vi "State_Machine.vi"(8 "error in (no error)":errorcluster caption="entrée d'erreur (pas d'erreur)", 11 "Send_Frame en entrée":refnum<class "Zigbee_Send_Command_UART.lvclass">) -> (0 "error out":errorcluster caption="sortie d'erreur", 2 "Json_String":string, 3 "Send_Frame en sortie":refnum<class "Zigbee_Send_Command_UART.lvclass">)   [LabVIEW 2020, in "Library Test.lvlib" / "Zigbee_Send_Command_UART.lvclass"]
uses:
  Zigbee_Send_Command_UART.lvclass
  Commun VI/TypeDef/Liste Error.ctl
  Zigbee_Send_Command_UART.lvclass/Zigbee_Send_Command_UART.ctl
  Commun VI/Library Commun.lvlib
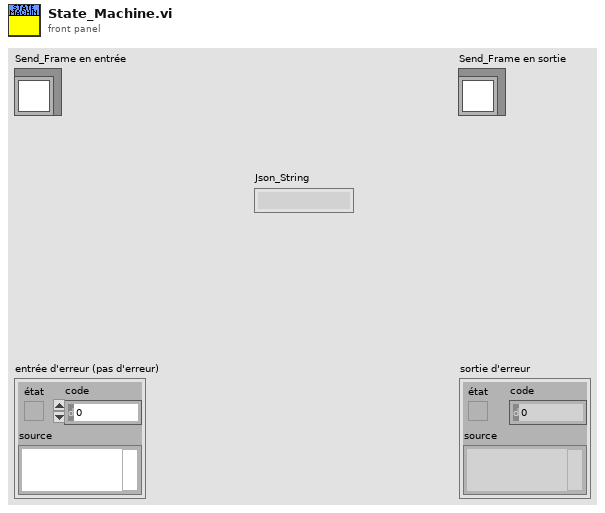
[diagram p1: front panel]
types:
  T1 = enum16{"Empty port", "Send Frame", "Wait Return", "Check End", "End"}
  T2 = typedef "Library Commun.lvlib/Liste Error.ctl" = enum16{"Firebase Driver - Get Document", "Firebase Driver - Get Document With Where", "Firebase Driver - Delete Document", "Firebase Driver - Set Document", "Firebase Driver - Update Document", "Firebase Altyor - Search Document Bench", "Firebase Altyor - Class Not in Firebase", "Spectrum_Analyser - Timeout", "Relay Board - Qty Relay", "DIO - Pb Funtion", "Power_Supply - Peripherical not find", "Mutimeter - Peripherical not find", "Instrument - Function Not Used", "Instrument - Instrument name not specified", "Instrument - Allready Initialised", "Instrument - TimeOut", "Instrument - the instrument must be Initialise before", "Instrument - Frame Not received", "Instrument - Frame Nok", "Test - Initialise the File_for_Save", "Test - Timeout", "Test - Cmd Error", "FGV - Variable ", "BDD FireBase - Define Class", "SN - Class Not Define"}
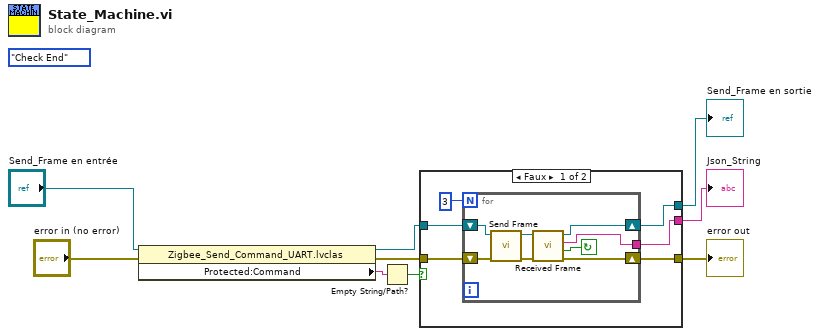
[diagram p0: block diagram]
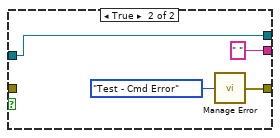
[diagram p2: hidden frame]
diagram:
  (unwired) T1."Check End"
  n1 = property class="Zigbee_Send_Command_UART.lvclas"(reference="Send_Frame en entrée", error in="error in (no error)") -> (reference out=w8:refnum<class "Zigbee_Send_Command_UART.lvclass">, error out=w7:errorcluster, "Protected:Command"=w4:string)
  n2 = Empty String/Path?(string/path=w4) -> (empty?=w3:bool)
  n3 = case shown="Faux" w3 {
    tunnel: [w13 w25] -> w2
    tunnel: w8 -> [w15 w25]
    tunnel: w7 -> [w14 _]
    tunnel: [w12 w27] -> w5
    tunnel: [w10 " " ("Frame read")] -> w1
    frame False {
      n4 = for {
        N: 3 -> [_]
        shift-right: [w20] -> w13
        shift-left: w15 -> [w23]
        shift-right: [w18] -> w12
        shift-left: w14 -> [w22]
        tunnel: [w16] -> w10
        stop <- w17 continue-if-true
        n5 = call-dynamic "Send Frame.vi"("entrée d'erreur (pas d'erreur)"=w22, "Send_Frame en entrée"=w23) -> ("sortie d'erreur"=w19:errorcluster, "Send_Frame en sortie"=w21:refnum<class "Zigbee_Send_Command_UART.lvclass">)  [unwired: 8 in]
        n6 = call-dynamic "Received Frame.vi"("entrée d'erreur (pas d'erreur)"=w19, "Send_Frame en entrée"=w21) -> ("sortie d'erreur"=w18:errorcluster, "Send again"=w17:bool, "Frame read"=w16:string, "Send_Frame en sortie"=w20:refnum<class "Zigbee_Send_Command_UART.lvclass">)  [unwired: 6 in]
      }
    }
    frame True {
      n7 = call "Manage Error.vi"("Code Erreur"=Liste_Error."Test - Cmd Error") -> ("error out"=w27:errorcluster)  [unwired: 14 in]
    }
  }
  "error out" <- w5
  "Send_Frame en sortie" <- w2
  "Json_String" <- w1
